vi "Powerlawfit_Ranjani_didntwork.vi"() -> ()   [LabVIEW 2020]
uses:
  <vilib>/Analysis/NI_AALPro.lvlib
panel:
  out "Residue of Vsd vs T":cluster{i32[], dbl[]}(graph)
  out "Power of Vsd vsT":cluster{i32[], dbl[]}(graph)
  in  "parameter bounds":T1={"amp min"=-inf, "amp max"=inf, "power min"=-inf, "power max"=inf, "offset min"=0.0, "offset max"=0.0}
  in  "A vs B":cluster{dbl[], dbl[]}[](graph)
  out "residue":dbl
  out "amplitude":dbl
  out "Fitoffset":dbl
  out "power":dbl
  in  "Offset":i32
  in  "length":i32
  out "Powerlaw fit":cluster{dbl[], dbl[]}[](graph)
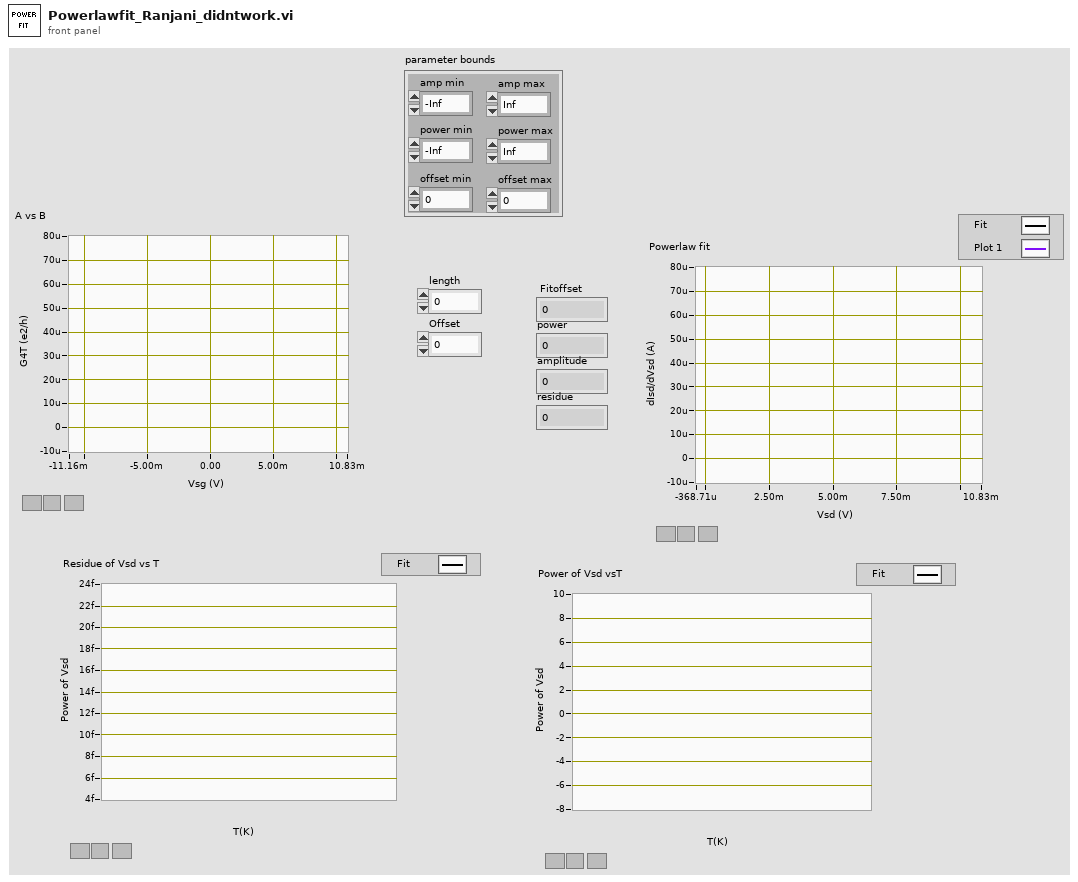
[diagram p1: front panel]
types:
  T1 = cluster{"amp min":dbl, "amp max":dbl, "power min":dbl, "power max":dbl, "offset min":dbl, "offset max":dbl}
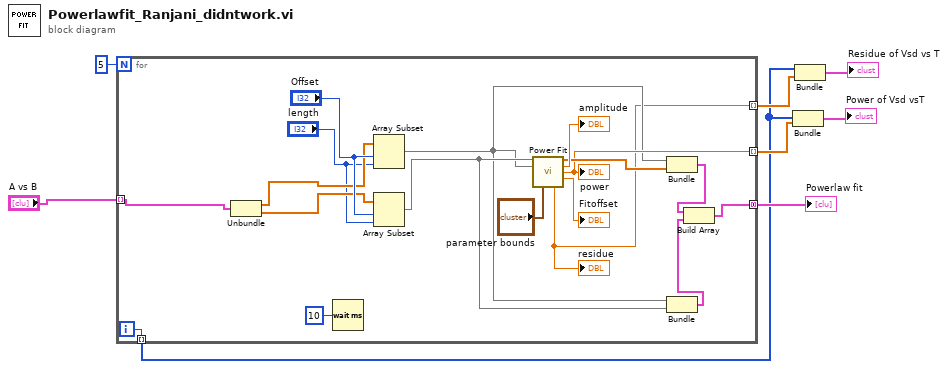
[diagram p0: block diagram]
diagram:
  n1 = for {
    N: 5 -> [_]
    tunnel: "A vs B" -> [w17] mode=indexing
    tunnel: [w13] -> w7 mode=concatenating
    tunnel: [w12] -> w5 mode=indexing
    tunnel: [w10] -> w2 mode=indexing
    tunnel: [w9] -> w3 mode=indexing
    i -> [w10]
    n2 = Unbundle(w17) -> (w20:dbl[], w19:dbl[])
    n3 = Wait (ms)(milliseconds to wait=u32 10) -> ()  [unwired: 1 out]
    n4 = Array Subset(array=w20, index="Offset", length="length") -> (w11:dbl[])
    n5 = Array Subset(array=w19, index="Offset", length="length") -> (w22:dbl[])
    n6 = call <vilib>:"Power Fit.vi"("Y"=w22, "X"=w11, "parameter bounds"="parameter bounds") -> ("Best Power Fit"=w21:dbl[], "amplitude"=→"amplitude":dbl, "power"=w12:dbl, "offset"=→"Fitoffset":dbl, "residue"=w9:dbl)  [unwired: 7 in, 1 out]
    "power" <- w12
    "residue" <- w9
    n7 = Bundle(w11, "Best Power Fit"=w21) -> (w15:cluster{dbl[], "Best Power Fit":dbl[]})  [unwired: 1 in]
    n8 = Bundle(w11, w22) -> (w14:cluster{dbl[], dbl[]})  [unwired: 1 in]
    n9 = Build Array(w15, w14) -> (w13:cluster{dbl[], "Best Power Fit":dbl[]}[])
  }
  "Powerlaw fit" <- w7
  n10 = Bundle(w2, w5) -> (→"Power of Vsd vsT":cluster{i32[], dbl[]})  [unwired: 1 in]
  n11 = Bundle(w2, w3) -> (→"Residue of Vsd vs T":cluster{i32[], dbl[]})  [unwired: 1 in]
